vi "Read Diagnostic PID Values.vi"(7 "Unit Address (1)":u8=1, 8 "error in (no error)":errorcluster, 11 "VISA resource name":refnum<visa-resource-name>) -> (0 "error out":errorcluster, 1 "Integral Output Contribution":i32, 2 "Proportional Output Contribution":i32, 3 "VISA resource name out":refnum<visa-resource-name>, 4 "Derivative Output Contribution":i32)   [LabVIEW 2014, in "Eurotherm 35xx Series.lvlib"]
doc: "This VI returns Diagnostic PID Values."
uses:
  <instrlib>/Eurotherm 35xx Series/Eurotherm 35xx Series.lvlib
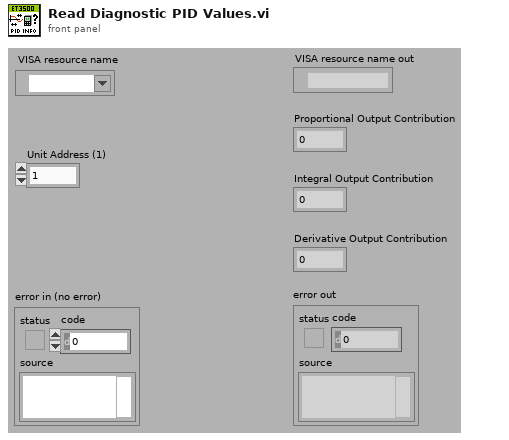
[diagram p1: front panel]
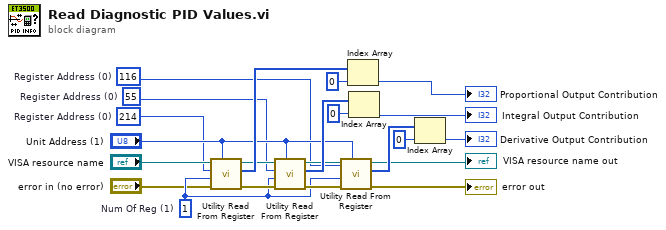
[diagram p0: block diagram]
diagram:
  w6 = 116  # Register Address (0)
  w5 = 55  # Register Address (0)
  w4 = 214  # Register Address (0)
  w12 = u16 1  # Num Of Reg (1)
  n1 = call <instrlib>:"Utility Read From Register.vi"("Unit Address (1)"="Unit Address (1)", "error in (no error)"="error in (no error)", "Num Of Reg (1)"=w12, "Register Address (0)"=w4, "VISA resource name"="VISA resource name") -> ("error out"=w13:errorcluster, "Data"=w22:i16[], "VISA resource name out"=w16:refnum<visa-resource-name>)  [unwired: 4 in]
  n2 = call <instrlib>:"Utility Read From Register.vi"("Unit Address (1)"="Unit Address (1)", "error in (no error)"=w13, "Num Of Reg (1)"=w12, "Register Address (0)"=w5, "VISA resource name"=w16) -> ("error out"=w14:errorcluster, "Data"=w19:i16[], "VISA resource name out"=w15:refnum<visa-resource-name>)  [unwired: 4 in]
  n3 = call <instrlib>:"Utility Read From Register.vi"("Unit Address (1)"="Unit Address (1)", "error in (no error)"=w14, "Num Of Reg (1)"=w12, "Register Address (0)"=w6, "VISA resource name"=w15) -> ("error out"=→"error out":errorcluster, "Data"=w18:i16[], "VISA resource name out"=→"VISA resource name out":refnum<visa-resource-name>)  [unwired: 4 in]
  n4 = Index Array(array=w22, index=0) -> (element=→"Proportional Output Contribution":i16)
  n5 = Index Array(array=w19, index=0) -> (element=→"Integral Output Contribution":i16)
  n6 = Index Array(array=w18, index=0) -> (element=→"Derivative Output Contribution":i16)
